vi "SV Limit Testing for Monitoring (1 Ch) (waveform) (DBL).vi"(7 "reset":bool, 9 "lower limit":dbl=-inf format="%.2f", 10 "upper limit":dbl=inf format="%.2f", 11 "signal in":waveform(dbl)) -> (1 "lower limit clearance":dbl format="%.6f", 2 "upper limit clearance":dbl format="%.6f", 3 "test passed?":bool, 5 "timestamp":timestamp format="%<%.6X\n%x>T")   [LabVIEW 2017]
doc: "Performs limit testing on waveforms, spectra, XY data, identified peaks, or scalar measurements. You can wire <B>output values</B> to a graph to view the limits, signal, and failures. Wire data to the<B> signal in</B> input to determine the polymorphic instance to use or manually select the instance."
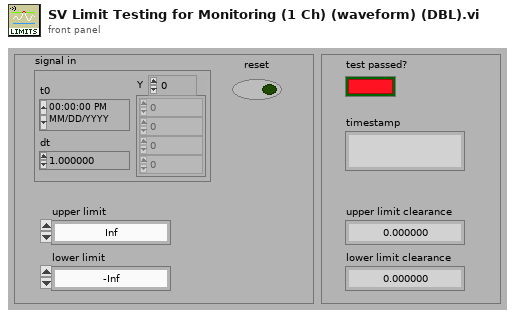
[diagram p1: front panel]
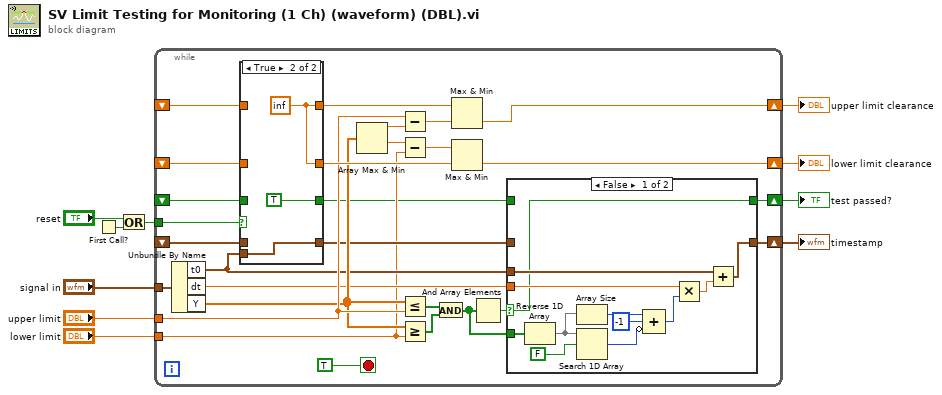
[diagram p0: block diagram]
diagram:
  n1 = First Call?() -> (First Call?: T/F=w2:bool)
  n2 = Or(x="reset", y=w2) -> (x .or. y?=w3:bool)
  n3 = while {
    tunnel: "signal in" -> [w38]
    tunnel: "upper limit" -> [w28]
    tunnel: "lower limit" -> [w17]
    shift-right: [w37] -> w7
    shift-left: _ -> [w34]
    shift-right: [w36] -> w6
    shift-left: _ -> [w32]
    shift-right: [w15] -> w5
    shift-left: _ -> [w30]
    shift-right: [w24] -> w1
    shift-left: _ -> [w29]
    tunnel: w3 -> [w35]
    stop <- TRUE stop-if-true
    n4 = Unbundle By Name(w38) -> ("t0"=w23:timestamp, "dt"=w22:dbl, "Y"=w27:dbl[])
    n5 = case shown="True" w35 {
      tunnel: w34 -> [w56 _]
      tunnel: [w56 w57] -> w33
      tunnel: w32 -> [w55 _]
      tunnel: [w55 w57] -> w31
      tunnel: w30 -> [w54 _]
      tunnel: [w54 TRUE] -> w16
      tunnel: w29 -> [w53 _]
      tunnel: [w53 w59] -> w25
      tunnel: w23 -> [_ w59]
      frame False {
      }
      frame True {
        w57 = inf
      }
    }
    n6 = Array Max & Min(array=w27) -> (max value=w14:dbl, min value=w13:dbl)  [unwired: 2 out]
    n7 = Subtract(x=w28, y=w14) -> (x-y=w12:dbl)
    n8 = Subtract(x=w13, y=w17) -> (x-y=w11:dbl)
    n9 = Less Or Equal?(x=w27, y=w28) -> (x <= y?=w19:bool[])
    n10 = Greater Or Equal?(x=w27, y=w17) -> (x >= y?=w18:bool[])
    n11 = And(x=w19, y=w18) -> (x .and. y?=w26:bool[])
    n12 = Max & Min(x=w33, y=w12) -> (min(x,y)=w37:dbl)  [unwired: 1 out]
    n13 = Max & Min(x=w11, y=w31) -> (min(x,y)=w36:dbl)  [unwired: 1 out]
    n14 = And Array Elements(Boolean array=w26) -> (logical AND=w21:bool)
    n15 = case shown="False" w21 {
      selector: w21 -> [w39 _]
      tunnel: w26 -> [w49 _]
      tunnel: w25 -> [_ w52]
      tunnel: [w43 w52] -> w24
      tunnel: w23 -> [w44 _]
      tunnel: w22 -> [w40 _]
      tunnel: w16 -> [_ w51]
      tunnel: [w39 w51] -> w15
      frame False {
        n16 = Reverse 1D Array(array=w49) -> (reversed array=w48:bool[])
        n17 = Array Size(array=w48) -> (size(s)=w47:i32)
        n18 = Search 1D Array(1D array=w48, element=FALSE) -> (index of element=w45:i32)  [unwired: 1 in]
        n19 = Compound Arithmetic op=ADD(w47, -1 ("value"), invert w45) -> (w41:i32)
        n20 = Multiply(x=w40, y=w41) -> (x*y=w42:dbl)
        n21 = Add(x=w44, y=w42) -> (x+y=w43:timestamp)
      }
      frame True {
      }
    }
  }
  "test passed?" <- w5
  "upper limit clearance" <- w7
  "lower limit clearance" <- w6
  "timestamp" <- w1
